vi "DSF.Engine.Transceiver Thread.Error Handler.vi"(8 "error in (no error)":errorcluster, 10 "stop":bool, 11 "Transceiver Thread in":refnum<class "DSF.Engine.Transceiver Thread.lvclass">) -> (0 "error out":errorcluster, 2 "stop":bool, 3 "Transceiver Thread out":refnum<class "DSF.Engine.Transceiver Thread.lvclass">)   [LabVIEW 2017, in "Data Sharing Framework Engine.lvlib" / "DSF.Engine.Transceiver Thread.lvclass"]
uses:
  DSF.Engine.Transceiver Thread.lvclass
  DSF.Engine.Transceiver Thread.lvclass/DSF.Engine.Transceiver Thread.ctl
  Source/Data Sharing Framework Core/Engine/Interfaces/Transceiver Interface/Write Transceiver Error.vi
  Source/Data Sharing Framework Core/Engine/Interfaces/Transceiver Interface/Transceiver Interface.lvclass
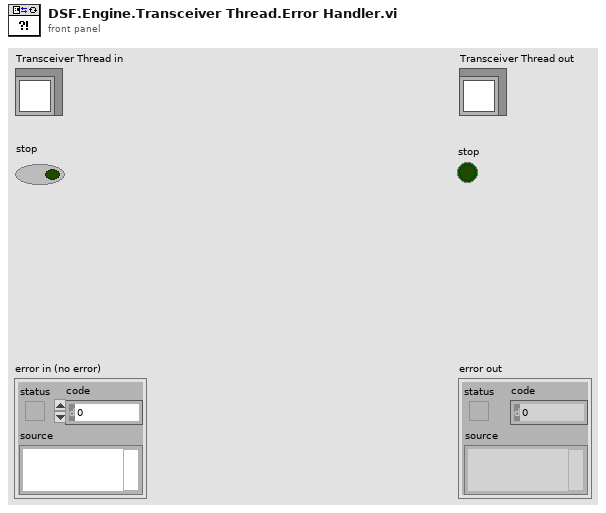
[diagram p1: front panel]
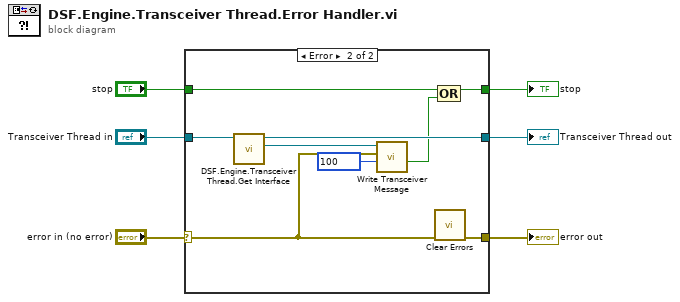
[diagram p0: block diagram]
diagram:
  n1 = case shown="Error" "error in (no error)" {
    selector: "error in (no error)" -> [w9 w10]
    tunnel: "stop" -> [w8 w13]
    tunnel: [w9 w11] -> w4
    tunnel: [w8 w12] -> w3
    tunnel: "Transceiver Thread in" -> [w7 w18]
    tunnel: [w7 w17] -> w1
    frame No Error {
    }
    frame Error {
      n2 = call "DSF.Engine.Transceiver Thread.Get Interface.vi"("Transceiver Thread in"=w18) -> ("Interface"=w16:refnum<class "Transceiver Interface.lvclass">, "Transceiver Thread out"=w17:refnum<class "DSF.Engine.Transceiver Thread.lvclass">)  [unwired: 9 in]
      n3 = call-poly "Write Transceiver Message.vi"("timeout in ms (0)"=100, "error"=w10, "Transceiver Interface in"=w16) -> ("timed out?"=w14:bool)  [unwired: 6 in, 2 out]
      n4 = call <vilib>:"Clear Errors.vi"("error in (no error)"=w10) -> ("error out"=w11:errorcluster)  [unwired: 5 in, 1 out]
      n5 = Compound Arithmetic op=OR(w13, w14) -> (w12:bool)
    }
  }
  "error out" <- w4
  "Transceiver Thread out" <- w1
  "stop" <- w3
